vi "controlOutput.vi"(7 "Set":bool, 8 "error in":errorcluster, 9 "enable output in":bool=TRUE, 10 "axis in":u8, 11 "connection ID":refnum<k5>) -> (0 "error out":errorcluster, 1 "enable output out":bool=TRUE, 2 "axis out":u8, 3 "connection ID":refnum<k5>)   [LabVIEW 2019]
panel:
  in  "Set Command":string="com.attocube.amc.control.setControlOutput"
  in  "Get Command":string="com.attocube.amc.control.getControlOutput"
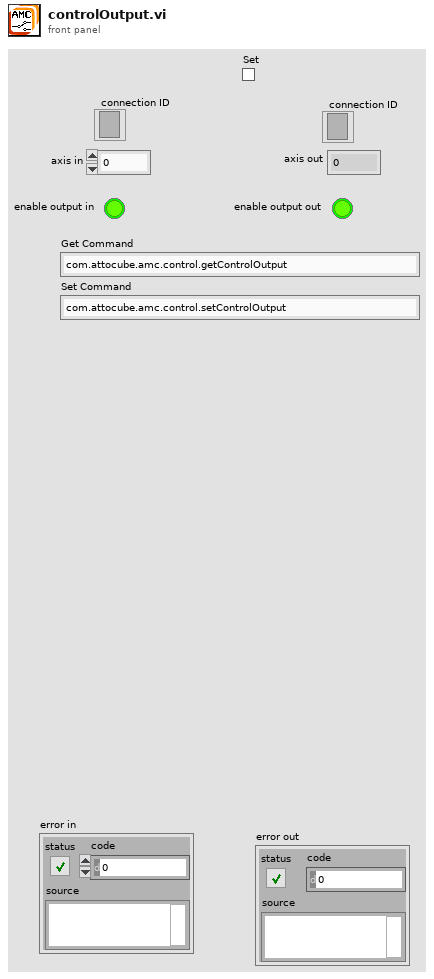
[diagram p1: front panel]
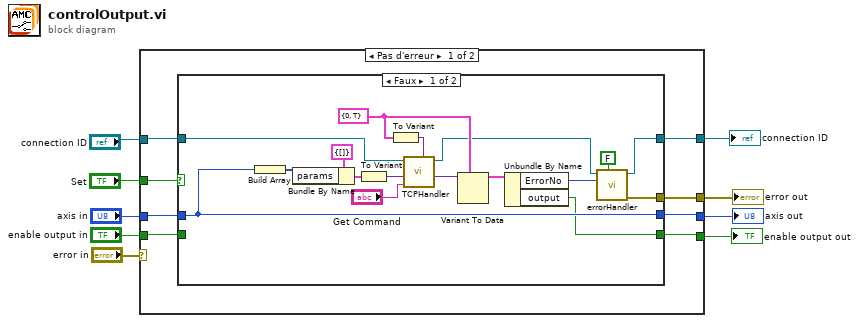
[diagram p0: block diagram]
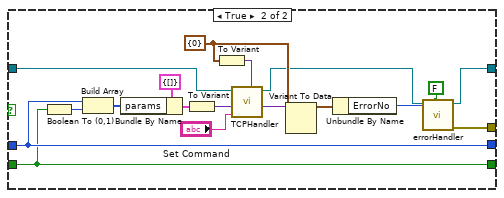
[diagram p2: hidden frame]
diagram:
  n1 = case shown="Pas d'erreur" "error in" {
    selector: "error in" -> [_ w56]
    tunnel: "axis in" -> [w15 w54]
    tunnel: [w10 w56] -> w1
    tunnel: [w14 w54] -> w8
    tunnel: "Set" -> [w11 _]
    tunnel: [w12 w55] -> w6
    tunnel: "enable output in" -> [w13 w55]
    tunnel: [w17 w53] -> w4
    tunnel: "connection ID" -> [w16 w53]
    frame No Error {
      n2 = case shown="Faux" w11 {
        tunnel: [w18 w35] -> w17
        tunnel: w16 -> [w23 w46]
        tunnel: w15 -> [w25 w44]
        tunnel: [w25 w44] -> w14
        tunnel: [w22 w43] -> w12
        tunnel: w13 -> [_ w43]
        tunnel: [w24 w39] -> w10
        frame False {
          w20 = cluster{"ErrorNo":i16, "output":bool} {"ErrorNo"=0, "output"=TRUE} ("input cluster")
          n3 = Build Array(w25) -> (w30:u8[])
          n4 = Bundle By Name(cluster=cluster{"params":i32[]} {"params"=[]} ("input cluster"), "params"=w30) -> (w31:cluster{"params":i32[]})
          n5 = To Variant(anything=w31) -> (Variant=w32:variant)
          n6 = To Variant(anything=w20) -> (Variant=w21:variant)
          n7 = call "TCPHandler.vi"("result Types"=w21, "method"="Get Command", "params"=w32, "connection ID"=w23) -> ("result"=w28:variant, "connection ID"=w19:refnum<k5>)  [unwired: 5 in, 1 out]
          n8 = Variant To Data(type=w20, Variant=w28) -> (data=w33:cluster{"ErrorNo":i16, "output":bool})  [unwired: 1 in, 1 out]
          n9 = Unbundle By Name(w33) -> ("ErrorNo"=w34:i16, "output"=w22:bool)
          n10 = call "errorHandler.vi"("show popup"=FALSE, "error number"=w34, "connection ID"=w19) -> ("error out"=w24:errorcluster, "connection ID"=w18:refnum<k5>)  [unwired: 7 in]
        }
        frame True {
          w37 = cluster{"ErrorNo":i16} {"ErrorNo"=0} ("input cluster")
          n11 = Boolean To (0,1)(Boolean=w43) -> (0, 1=w50:i16)
          n12 = Build Array(w44, w50) -> (w48:i16[])
          n13 = Bundle By Name(cluster=cluster{"params":i32[]} {"params"=[]} ("input cluster"), "params"=w48) -> (w47:cluster{"params":i32[]})
          n14 = To Variant(anything=w47) -> (Variant=w45:variant)
          n15 = To Variant(anything=w37) -> (Variant=w38:variant)
          n16 = call "TCPHandler.vi"("result Types"=w38, "method"="Set Command", "params"=w45, "connection ID"=w46) -> ("result"=w51:variant, "connection ID"=w36:refnum<k5>)  [unwired: 5 in, 1 out]
          n17 = Variant To Data(type=w37, Variant=w51) -> (data=w41:cluster{"ErrorNo":i16})  [unwired: 1 in, 1 out]
          n18 = Unbundle By Name(w41) -> ("ErrorNo"=w40:i16)
          n19 = call "errorHandler.vi"("show popup"=FALSE, "error number"=w40, "connection ID"=w36) -> ("error out"=w39:errorcluster, "connection ID"=w35:refnum<k5>)  [unwired: 7 in]
        }
      }
    }
    frame Error {
    }
  }
  "error out" <- w1
  "axis out" <- w8
  "enable output out" <- w6
  "connection ID" <- w4
